vi "Test 1.vi"() -> ()   [LabVIEW 2021, in "Hex Viewer.lvclass"]
uses:
  Hex Viewer.lvclass
  Memory/Memory.lvclass/Memory.ctl
  Memory/Memory.lvclass
panel:
  in  "stop":bool
  in  "Address":u16 format="%.0x"
  in  "Table Control":string[][](table)
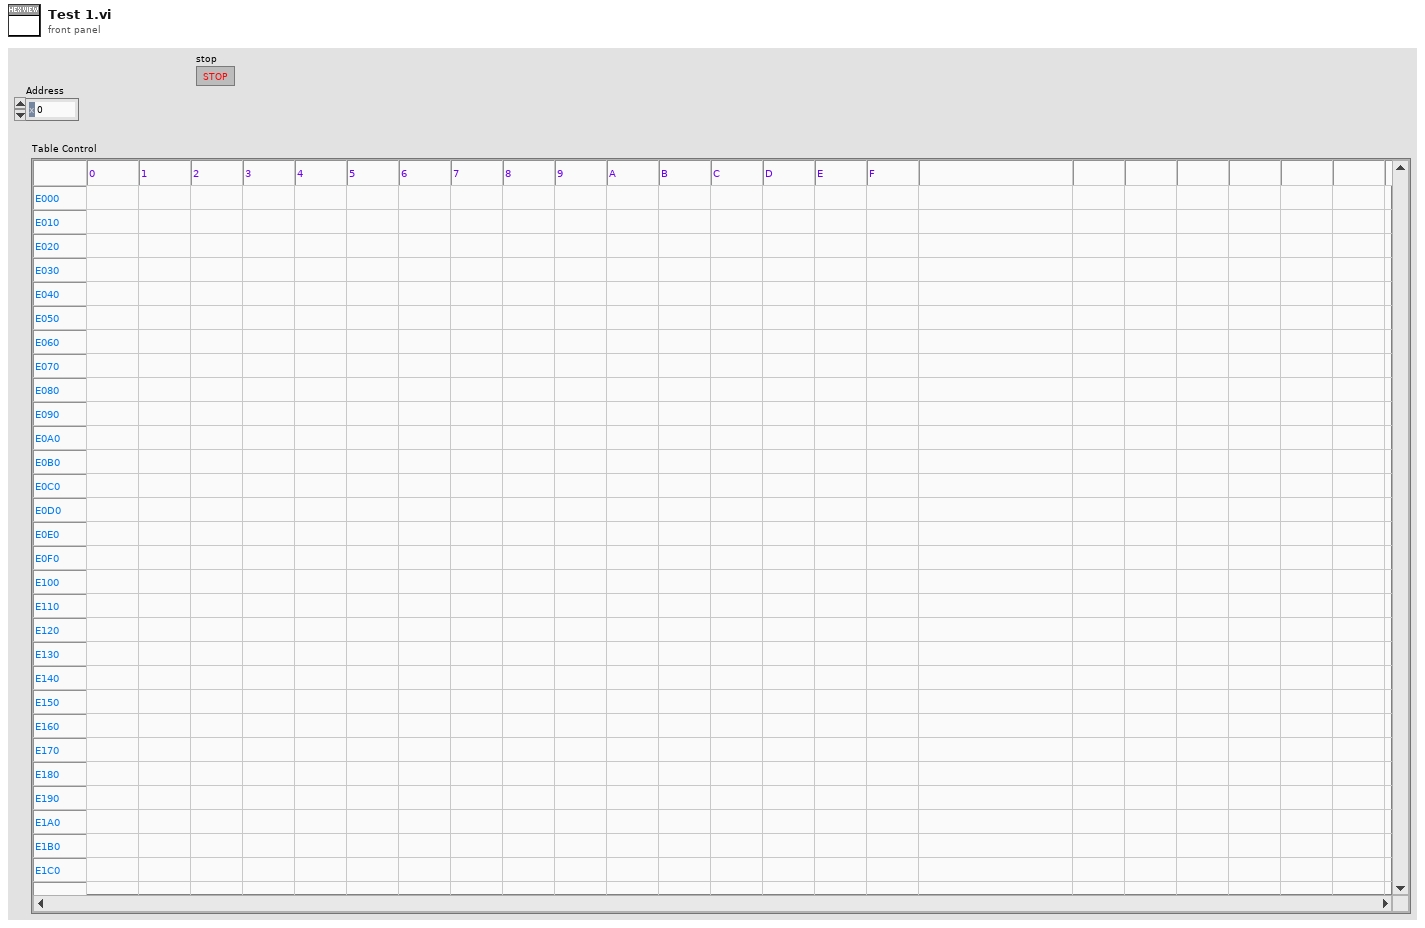
[diagram p1: front panel]
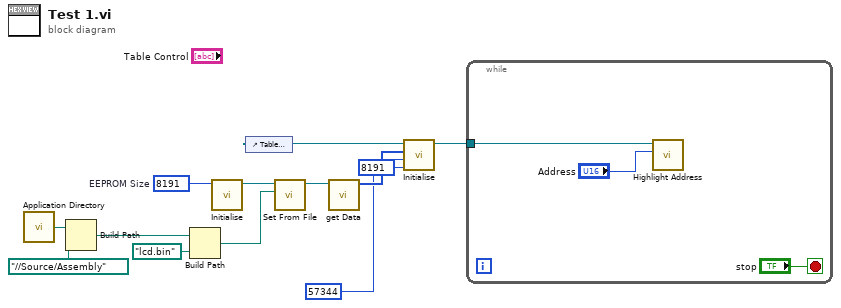
[diagram p0: block diagram]
diagram:
  w5 = u16 8191  # EEPROM Size
  n1 = call <vilib>:"Application Directory.vi"() -> ("Application Directory"=w10:path)
  n2 = Build Path(base path=w10, name or relative path=path "../../Source/Assembly" ("ROM")) -> (appended path=w8:path)
  n3 = Build Path(base path=w8, name or relative path=path "lcd.bin") -> (appended path=w6:path)
  n4 = call "Initialise.vi"("Size"=w5) -> ("Memory out"=w11:refnum<class "Memory.lvclass">)  [unwired: 10 in]
  n5 = control-ref of="Table Control"() -> (w13:refnum<vi>)
  n6 = call "Set From File.vi"("Memory binary"=w6, "Memory in"=w11) -> ("Memory out"=w12:refnum<class "Memory.lvclass">)  [unwired: 8 in, 1 out]
  n7 = call "get Data.vi"("Memory in"=w12) -> ("Data"=w4:u8[])  [unwired: 10 in]
  n8 = call "Initialise.vi"("Size"=u16 8191, "Offset"=u16 57344, "Data"=w4, "Table"=w13) -> ("Hex Viewer"=w3:refnum<class "Hex Viewer.lvclass">)  [unwired: 7 in]
  n9 = while {
    tunnel: w3 -> [w16]
    stop <- "stop" stop-if-true
    n10 = call "Highlight Address.vi"("Address"="Address", "Hex Viewer in"=w16) -> ()  [unwired: 10 in]
  }
